vi "Format JSON Array Text.vi"(6 "Pretty Print?":bool, 8 "error in (no error)":errorcluster, 10 "Array of JSON Text":string[](array[string])) -> (0 "error out":errorcluster, 3 "<JSON>":string)   [LabVIEW 2017, in "JSONtext.lvlib"]
uses:
  JSONtext.lvlib
  <vilib>/JDP Science/JDP Science Common Utilities/JDP Utility.lvlib
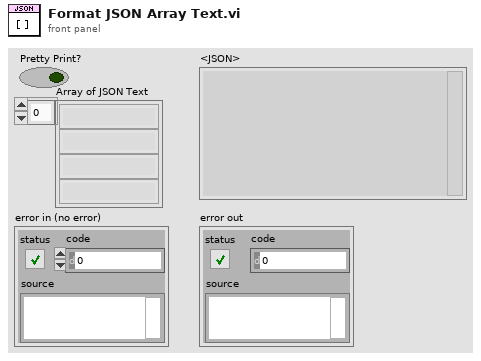
[diagram p1: front panel]
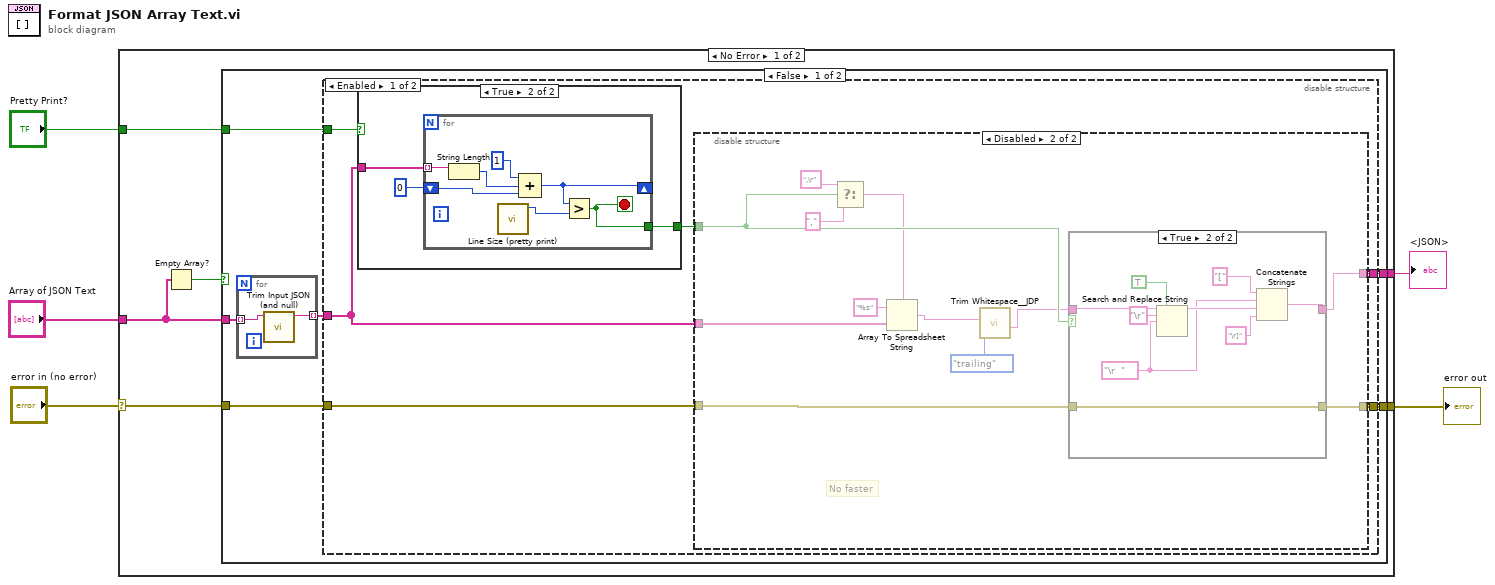
[diagram p0: block diagram]
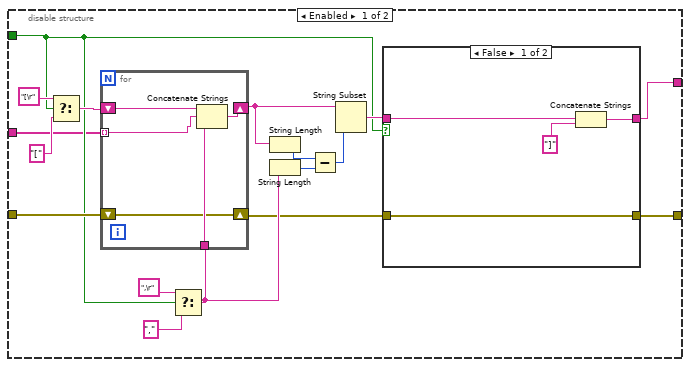
[diagram p2: hidden frame]
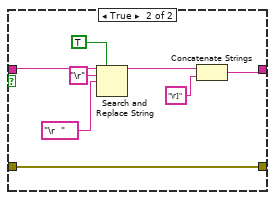
[diagram p3: hidden frame]
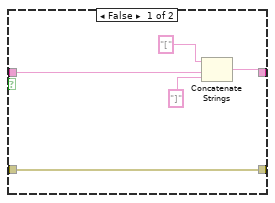
[diagram p4: hidden frame]
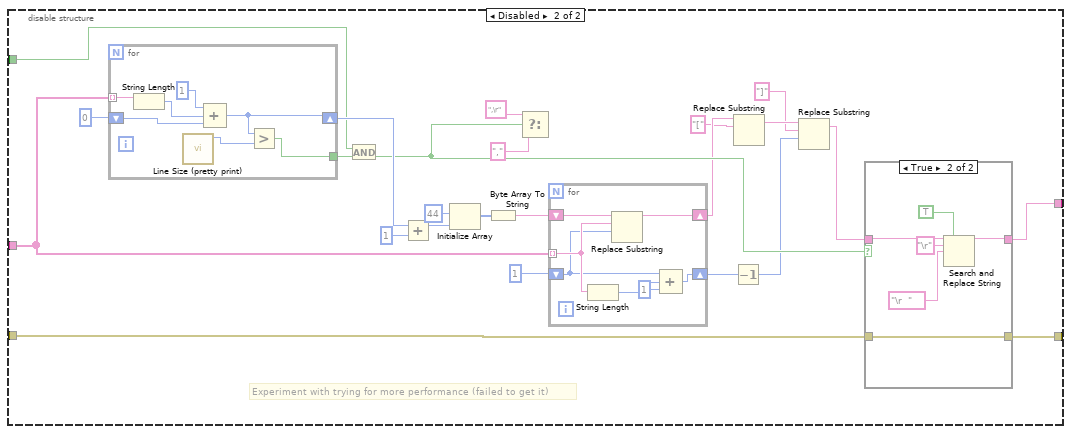
[diagram p6: hidden frame]
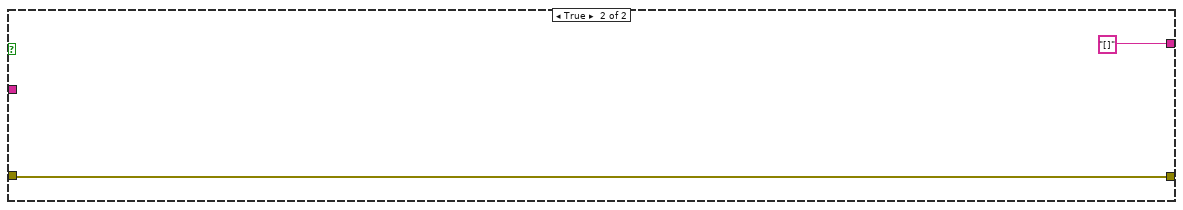
[diagram p8: hidden frame]
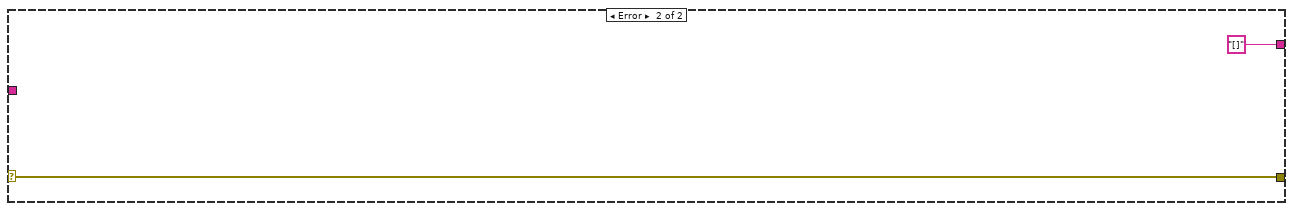
[diagram p9: hidden frame]
diagram:
  n1 = case shown="No Error" "error in (no error)" {
    selector: "error in (no error)" -> [w10 w145]
    tunnel: [w11 "[]" ("t")] -> w5
    tunnel: "Pretty Print?" -> [w9 _]
    tunnel: "Array of JSON Text" -> [w7 _]
    tunnel: [w8 w145] -> w1
    frame No Error {
      n2 = Empty Array?(array=w7) -> (empty?=w6:bool)
      n3 = case shown="False" w6 {
        tunnel: [w16 "[]" ("t")] -> w11
        tunnel: w10 -> [w17 w142]
        tunnel: w9 -> [w15 _]
        tunnel: [w13 w142] -> w8
        tunnel: w7 -> [w12 _]
        frame False {
          n4 = for {
            tunnel: w12 -> [w141] mode=indexing
            tunnel: [w140] -> w14 mode=indexing
            n5 = call "Trim Input JSON (and null).vi"("JSON Input"=w141) -> ("<JSON>"=w140:string)  [unwired: 10 in]
          }
          n6 = disable-structure shown="Enabled" {
            disable-tunnel: w17 -> [w23 w117]
            disable-tunnel: [w22 w116] -> w16
            disable-tunnel: w15 -> [w21 w109]
            disable-tunnel: w14 -> [w19 w114]
            disable-tunnel: [w18 w113] -> w13
            frame Enabled {
              n7 = case shown="True" w21 {
                tunnel: w19 -> [_ w86]
                tunnel: [_ w84] -> w20
                frame False {
                }
                frame True {
                  n8 = for {
                    tunnel: w86 -> [w93] mode=indexing
                    shift-right: [w91] -> _
                    shift-left: 0 -> [w92]
                    tunnel: [w90] -> w84
                    stop <- w90 stop-if-true
                    n9 = String Length(string=w93) -> (length=w89:i32)
                    n10 = call "Line Size (pretty print).vi"() -> ("Line Size"=w88:i32)  [unwired: 11 in]
                    n11 = Compound Arithmetic op=ADD(1 ("value"), w89, w92) -> (w91:i32)
                    n12 = Greater?(x=w91, y=w88) -> (0:w90:bool)
                  }
                }
              }
              n13 = disable-structure shown="Disabled" {
                disable-tunnel: w23 -> [w40 w58]
                disable-tunnel: [w39 w69] -> w22
                disable-tunnel: w20 -> [w27 w66]
                disable-tunnel: w19 -> [w26 w64]
                disable-tunnel: [w24 w65] -> w18
                frame Enabled {
                  n14 = Select(t="[\r", s=w27, f="[") -> (s? t:f=w34:string)
                  n15 = Select(t=",\r" ("string"), s=w27, f="," ("string")) -> (s? t:f=w38:string)
                  n16 = for {
                    tunnel: w26 -> [w54] mode=indexing
                    shift-right: [w57] -> w30
                    shift-left: w34 -> [w56]
                    shift-right: [w53] -> w25
                    shift-left: w40 -> [w53]
                    tunnel: w38 -> [w55]
                    n17 = Concatenate Strings(w56, w54, w55) -> (w57:string)
                  }
                  n18 = String Length(string=w30) -> (length=w31:i32)
                  n19 = String Length(string=w38) -> (length=w32:i32)
                  n20 = Subtract(x=w31, y=w32) -> (x-y=w33:i32)
                  n21 = String Subset(string=w30, length (rest)=w33) -> (substring=w35:string)  [unwired: 1 in]
                  n22 = case shown="False" w27 {
                    tunnel: w35 -> [w42 w48]
                    tunnel: [w43 w49] -> w39
                    tunnel: w25 -> [w41 w45]
                    tunnel: [w41 w45] -> w24
                    frame False {
                      n23 = Concatenate Strings(w42, "]" ("substring (\"\")")) -> (w43:string)
                    }
                    frame True {
                      n24 = Search and Replace String(replace all?=TRUE ("replace all? (F)"), input string=w48, search string="\r", replace string="\r  " ("search string")) -> (result string=w50:string)  [unwired: 4 in, 3 out]
                      n25 = Concatenate Strings(w50, "\r]" ("search string")) -> (w49:string)
                    }
                  }
                }
                frame Disabled {
                  # "No faster"
                  n26 = Select(t=",\r" ("string"), s=w66, f="," ("string")) -> (s? t:f=w63:string)
                  n27 = Array To Spreadsheet String(delimiter (Tab)=w63, array=w64, 3:"%s" ("format string")) -> (spreadsheet string=w62:string)
                  n28 = call <vilib>:"Trim Whitespace__JDP.vi"("Remove (leading and trailing)"=enum16{"leading", "trailing", "both"}."trailing", "String in"=w62) -> ("String out"=w60:string)  [unwired: 5 in]
                  n29 = case shown="True" w66 {
                    tunnel: w60 -> [w72 w79]
                    tunnel: [w73 w80] -> w69
                    tunnel: w58 -> [w71 w77]
                    tunnel: [w71 w77] -> w65
                    frame False {
                      n30 = Concatenate Strings("[", w72, "]" ("substring (\"\")")) -> (w73:string)
                    }
                    frame True {
                      w76 = "\r  " ("search string")
                      n31 = Search and Replace String(replace all?=TRUE ("replace all? (F)"), input string=w79, search string="\r", replace string=w76) -> (result string=w81:string)  [unwired: 4 in, 3 out]
                      n32 = Concatenate Strings("[", w76, w81, "\r]" ("search string")) -> (w80:string)
                    }
                  }
                }
              }
            }
            frame Disabled {
              # "Experiment with trying for more performance (failed to get it)"
              n33 = for {
                tunnel: w114 -> [w139] mode=indexing
                shift-right: [w137] -> w112
                shift-left: 0 -> [w138]
                tunnel: [w136] -> w115
                n34 = String Length(string=w139) -> (length=w135:i32)
                n35 = call "Line Size (pretty print).vi"() -> ("Line Size"=w134:i32)  [unwired: 11 in]
                n36 = Compound Arithmetic op=ADD(1 ("value"), w135, w138) -> (w137:i32)
                n37 = Greater?(x=w137, y=w134) -> (0:w136:bool)
              }
              n38 = And(x=w109, y=w115) -> (x .and. y?=w110:bool)
              n39 = Add(x=w112, y=1) -> (x+y=w102:i32)
              n40 = Initialize Array(u8 44, w102) -> (w105:u8[])
              n41 = Byte Array To String(unsigned byte array=w105) -> (string=w104:string)
              n42 = Select(t=",\r" ("string"), s=w110, f="," ("string")) -> ()  [unwired: 1 out]
              n43 = for {
                tunnel: w114 -> [w122] mode=indexing
                shift-right: [w123] -> w100
                shift-left: w104 -> [w124]
                shift-right: [w118] -> w96
                shift-left: 1 -> [w121]
                n44 = String Length(string=w122) -> (length=w120:i32)
                n45 = Replace Substring(3:w121, 4:w122, 5:w124) -> (1:w123:string)  [unwired: 1 in, 1 out]
                n46 = Compound Arithmetic op=ADD(w121, w120, 1 ("value")) -> (w118:i32)
              }
              n47 = Decrement(x=w96) -> (x-1=w94:i32)
              n48 = Replace Substring(4:"[", 5:w100) -> (1:w98:string)  [unwired: 2 in, 1 out]
              n49 = Replace Substring(3:w94, 4:"]" ("search string"), 5:w98) -> (1:w95:string)  [unwired: 1 in, 1 out]
              n50 = case shown="True" w110 {
                tunnel: w95 -> [w125 w130]
                tunnel: w117 -> [w126 w129]
                tunnel: [w126 w129] -> w113
                tunnel: [w125 w127] -> w116
                frame False {
                }
                frame True {
                  n51 = Search and Replace String(replace all?=TRUE ("replace all? (F)"), input string=w130, search string="\r", replace string="\r  " ("search string")) -> (result string=w127:string)  [unwired: 4 in, 3 out]
                }
              }
            }
          }
        }
        frame True {
        }
      }
    }
    frame Error {
    }
  }
  "<JSON>" <- w5
  "error out" <- w1
